vi "enumerateStaticDependencies.vi"(8 "error in (no error)":errorcluster, 11 "SMO.Example":refnum<class "SMO.Example.lvclass">) -> (0 "error out":errorcluster, 2 "Static Dependencies":refnum<class "Dependency.lvclass">[](array[class]), 3 "SMO.Example out":refnum<class "SMO.Example.lvclass">)   [LabVIEW 2013, in "SMO.Example.lvclass"]
uses:
  SMO.Example.lvclass
  Dependency/Dependency.lvclass
  Typedefs/Dependencies--Cluster.ctl
  SMO.UI/SMO.UI.lvclass
  SMO/SMO.lvclass
panel:
  # "For instructions on how to use the JKI State Machine Objects, examples and video tutorials, visit:\nhttp://jki.net/state-machine-objects/\n\nJKI State Machine Objects™\nhttp://jki.net/state-machine-objects/\nCopyright (C) 2005-2015, JKI <info@jki.net>\nALL RIGHTS RESERVED"
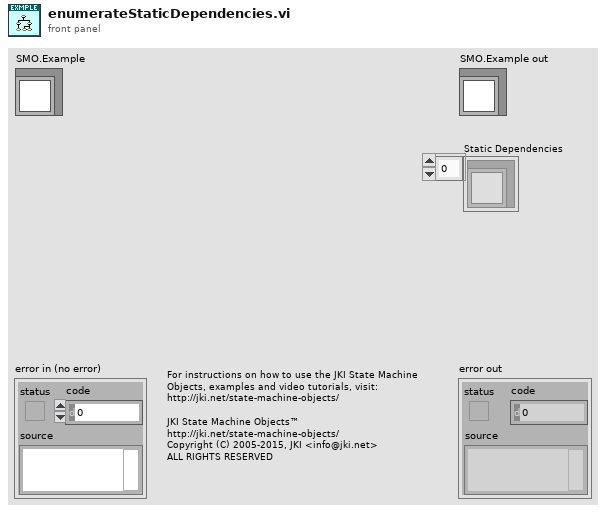
[diagram p1: front panel]
types:
  T1 = typedef "SMO.Example.lvclass/Dependencies--Cluster.ctl" = cluster{"About":refnum<class "SMO.UI.lvclass">}
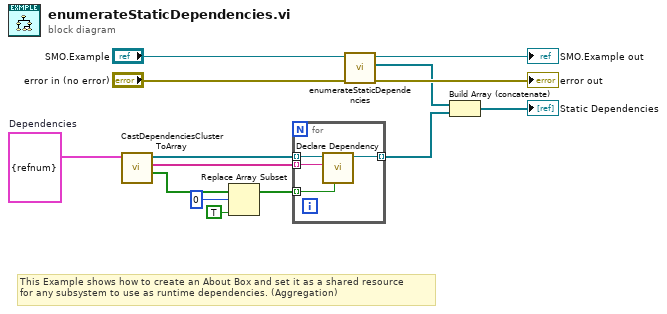
[diagram p0: block diagram]
diagram:
  w8 = T1 {"About"=refnum}  # Dependencies
  # "This Example shows how to create an About Box and set it as a shared resource\nfor any subsystem to use as runtime dependencies. (Aggregation)"
  n1 = call "CastDependenciesClusterToArray.vi"("Dependencies Cluster"=w8) -> ("Shared Resources"=w4:bool[], "Dependencies Names"=w9:string[], "Dependencies Array"=w10:refnum<class "SMO.lvclass">[])  [unwired: 8 in]
  n2 = Replace Array Subset(array=w4, new element=TRUE ("Shared Resource (F)"), index=0) -> (w3:bool[])
  n3 = for {
    tunnel: [w18] -> w7 mode=indexing
    tunnel: w10 -> [w17] mode=indexing
    tunnel: w9 -> [w16] mode=indexing
    tunnel: w3 -> [w15] mode=indexing
    n4 = call "Declare Dependency.vi"("Shared Resource (F)"=w15, "Name"=w16, "Type"=w17) -> ("Dependency out"=w18:refnum<class "Dependency.lvclass">)  [unwired: 7 in, 1 out]
  }
  n5 = call-parent "enumerateStaticDependencies.vi"("error in (no error)"="error in (no error)", "SMO"="SMO.Example") -> ("error out"=→"error out":errorcluster, "Static Dependencies"=w2:refnum<class "Dependency.lvclass">[], "SMO out"=→"SMO.Example out":refnum<class "SMO.Example.lvclass">)  [unwired: 7 in]
  n6 = Build Array (concatenate)(w2, w7) -> (→"Static Dependencies":refnum<class "Dependency.lvclass">[])
